vi "set_query mode.vi"(8 "error in (no error)":errorcluster, 9 "Mode Selector":enum16{"Withdraw", "Infuse"}(ring), 10 "Query?":bool, 11 "VISA resource name":refnum<visa-resource-name>) -> (0 "error out":errorcluster, 1 "Mode":string, 2 "Infuse?":bool=TRUE, 3 "VISA resource name out":refnum<visa-resource-name>, 5 "Withdraw?":bool=TRUE)   [LabVIEW 2016]
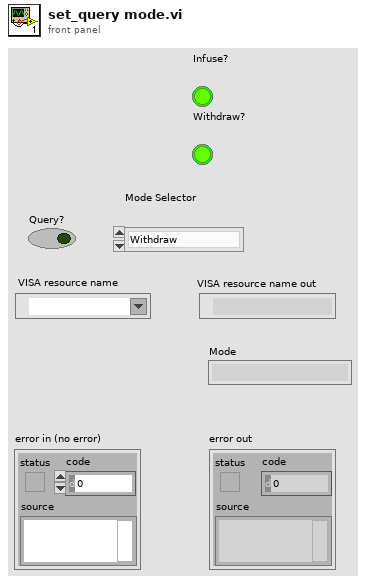
[diagram p1: front panel]
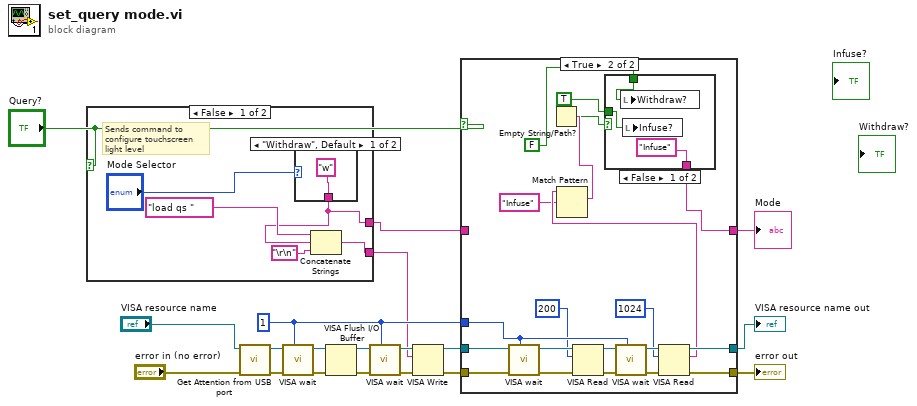
[diagram p0: block diagram]
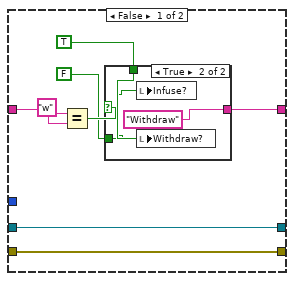
[diagram p2: hidden frame]
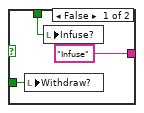
[diagram p3: hidden frame]
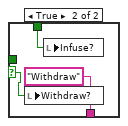
[diagram p4: hidden frame]
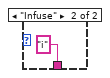
[diagram p5: hidden frame]
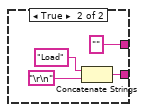
[diagram p6: hidden frame]
diagram:
  w5 = u32 1 ("milliseconds to wait")
  n1 = case shown="False" "Query?" {
    tunnel: [w22 w28] -> w4
    tunnel: [w20 ""] -> w1
    frame False {
      # "Sends command to configure touchscreen light level"
      n2 = case shown="\"Withdraw\", Default" "Mode Selector" {
        tunnel: ["w" "i"] -> w20
        frame "Withdraw", Default {
        }
        frame "Infuse" {
        }
      }
      n3 = Concatenate Strings("load qs " ("command"), w20, "\r\n") -> (w22:string)
    }
    frame True {
      n4 = Concatenate Strings("Load" ("command"), "\r\n") -> (w28:string)
    }
  }
  n5 = call "Get Attention from USB port.vi"("error in (no error)"="error in (no error)", "VISA resource name"="VISA resource name") -> ("error out"=w16:errorcluster, "VISA resource name out"=w17:refnum<visa-resource-name>)  [unwired: 8 in]
  n6 = call <userlib>:"VISA wait.vi"("VISA resource name"=w17, "error in (no error)"=w16, "milliseconds to wait"=w5) -> ("VISA resource name out"=w14:refnum<visa-resource-name>, "error out"=w15:errorcluster)  [unwired: 6 in]
  n7 = VISA Flush I/O Buffer(VISA resource name=w14, error in (no error)=w15) -> (VISA resource name out=w9:refnum<visa-resource-name>, error out=w8:errorcluster)  [unwired: 1 in]
  n8 = call <userlib>:"VISA wait.vi"("VISA resource name"=w9, "error in (no error)"=w8, "milliseconds to wait"=w5) -> ("VISA resource name out"=w7:refnum<visa-resource-name>, "error out"=w6:errorcluster)  [unwired: 6 in]
  n9 = VISA Write(VISA resource name=w7, write buffer=w4, error in (no error)=w6) -> (VISA resource name out=w13:refnum<visa-resource-name>, error out=w12:errorcluster)  [unwired: 1 out]
  n10 = case shown="True" "Query?" {
    tunnel: w13 -> [w38 w64]
    tunnel: w12 -> [w37 w63]
    tunnel: [w38 w56] -> w11
    tunnel: [w37 w55] -> w10
    tunnel: w5 -> [_ w54]
    tunnel: [w33 w47] -> w2
    tunnel: w1 -> [w36 _]
    frame False {
      n11 = Equal?(x=w36, y="w") -> (x = y?=w34:bool)
      n12 = case shown="True" w34 {
        tunnel: ["Infuse" ("read buffer") "Withdraw" ("read buffer")] -> w33
        tunnel: TRUE -> [w40 w43]
        tunnel: FALSE -> [w39 w42]
        frame False {
          n13 = local write "Withdraw?"(w39) -> ()
          n14 = local write "Infuse?"(w40) -> ()
        }
        frame True {
          n15 = local write "Infuse?"(w42) -> ()
          n16 = local write "Withdraw?"(w43) -> ()
        }
      }
    }
    frame True {
      n17 = call <userlib>:"VISA wait.vi"("VISA resource name"=w64, "error in (no error)"=w63, "milliseconds to wait"=w54) -> ("VISA resource name out"=w61:refnum<visa-resource-name>, "error out"=w62:errorcluster)  [unwired: 6 in]
      n18 = VISA Read(VISA resource name=w61, byte count=u32 200, error in (no error)=w62) -> (VISA resource name out=w60:refnum<visa-resource-name>, error out=w59:errorcluster)  [unwired: 2 out]
      n19 = call <userlib>:"VISA wait.vi"("VISA resource name"=w60, "error in (no error)"=w59, "milliseconds to wait"=w54) -> ("VISA resource name out"=w57:refnum<visa-resource-name>, "error out"=w58:errorcluster)  [unwired: 6 in]
      n20 = VISA Read(VISA resource name=w57, byte count=u32 1024, error in (no error)=w58) -> (VISA resource name out=w56:refnum<visa-resource-name>, read buffer=w51:string, error out=w55:errorcluster)  [unwired: 1 out]
      n21 = Match Pattern(string=w51, regular expression="Infuse") -> (match substring=w49:string)  [unwired: 1 in, 3 out]
      n22 = Empty String/Path?(string/path=w49) -> (empty?=w48:bool)
      n23 = case shown="False" w48 {
        selector: w48 -> [_ w69]
        tunnel: ["Infuse" "Withdraw"] -> w47
        tunnel: TRUE -> [w66 _]
        tunnel: FALSE -> [w65 w68]
        frame False {
          n24 = local write "Withdraw?"(w65) -> ()
          n25 = local write "Infuse?"(w66) -> ()
        }
        frame True {
          n26 = local write "Withdraw?"(w69) -> ()
          n27 = local write "Infuse?"(w68) -> ()
        }
      }
    }
  }
  "VISA resource name out" <- w11
  "error out" <- w10
  "Mode" <- w2
